vi "Expectedtime.vi"(2 "N":dbl, 3 "I":dbl, 4 "Reference time":timestamp) -> (0 "Expected time":dbl, 1 "Elapsed time":dbl)   [LabVIEW 2019]
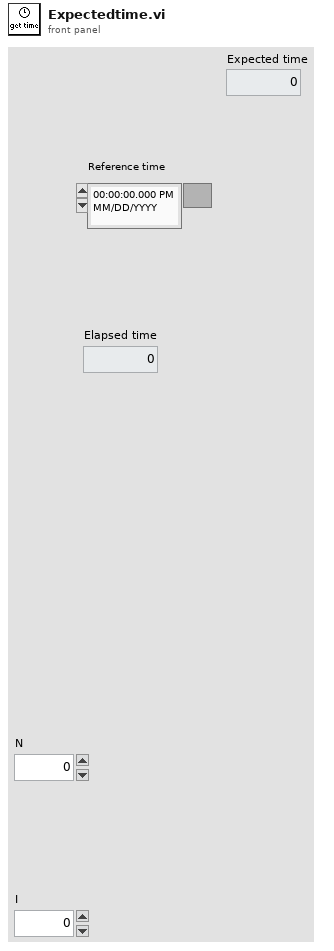
[diagram p1: front panel]
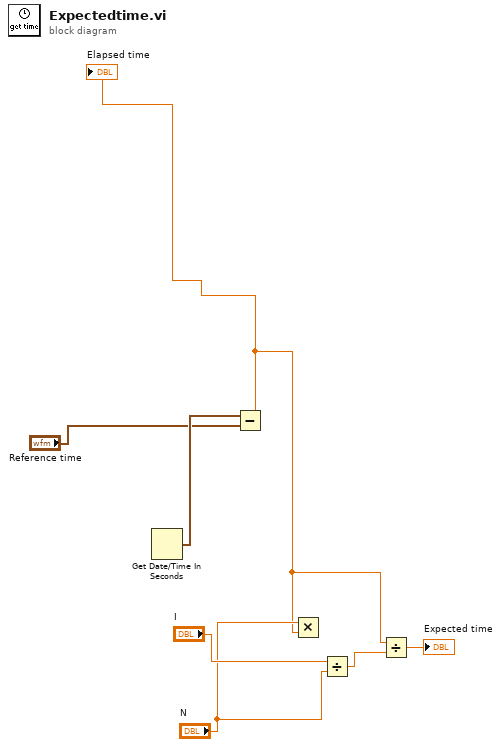
[diagram p0: block diagram]
diagram:
  n1 = Get Date/Time In Seconds() -> (seconds since 1Jan1904=w7:timestamp)
  n2 = Subtract(x=w7, y="Reference time") -> (x-y=w2:dbl)
  "Elapsed time" <- w2
  n3 = Multiply(x="N", y=w2) -> ()  [unwired: 1 out]
  n4 = Divide(x="I", y="N") -> (x/y=w4:dbl)
  n5 = Divide(x=w2, y=w4) -> (x/y=→"Expected time":dbl)
